vi "Lab3_FSK.vi"() -> ()   [LabVIEW 2019]
uses:
  <vilib>/addons/Modulation/Digital/General/MT Generate Bits (Galois, PN Order).vi
  <vilib>/addons/Modulation/Digital/Support/Common/Validators/mod_Generate Bits Validate.vi
  <vilib>/addons/Modulation/Analog/support/mod_Set Error Source.vi
  <vilib>/addons/Modulation/Digital/Support/Common/Validators/mod_AWGN Validate.vi
  <vilib>/addons/Modulation/Digital/Impairments/subVIs/mod_createSeeds.vi
  <vilib>/addons/Modulation/Digital/Support/Common/Validators/mod_Validate Samples Per Symbol.vi
  <vilib>/addons/Modulation/Analog/support/Validators/mod_Validate Complex Waveform.vi
  <vilib>/addons/Modulation/Analog/support/Validators/mod_WFErrorHandler.vi
  <vilib>/addons/Modulation/Digital/General/subVIs/mod_Generate Bits PN Sequence.vi
  <vilib>/addons/Modulation/Digital/General/MT Generate FSK System Parameters(M).vi
  <vilib>/Analysis/1siggen.llb/Gaussian White Noise (obs 90).vi
  <vilib>/addons/Modulation/Analog/MT Upconvert Baseband (Real).vi
  <vilib>/express/express analysis/Spectral/Block/exnSpectralBlock spectral measurements RMS poly.vi
  <vilib>/express/express analysis/Spectral/Block/exnSpectralBlock spectral measurements RMS DDT.vi
  <vilib>/express/express analysis/Spectral/XNode/ExpressSpectralMeasurementsBlockNode.xnode
  <vilib>/addons/Modulation/niDMT.lvlib
  <vilib>/addons/Modulation/niAMT.lvlib
panel:
  in  "stop 2":bool
  in  "Tab Control":enum32{"FFR(RMS)", "Module Signal"}(tab)
  out "FFR(RMS)":dynamicdata(graph)
  out "Module Signal":cluster{"t0":dbl, "dt":dbl, "Y":dbl[]}(graph)
  in  "FSK Derivation":dbl format="%#_2p"
  in  "Symbol (HZ)":dbl format="%#_2p"
  in  "Carrier Freq(HZ)":dbl format="%#_2p"
  in  "M-FSK":u16(ring) items=["2"=2, "4"=4, "8"=8, "16"=16]
  in  "Eb/No(dB)":dbl
  in  "stop":bool
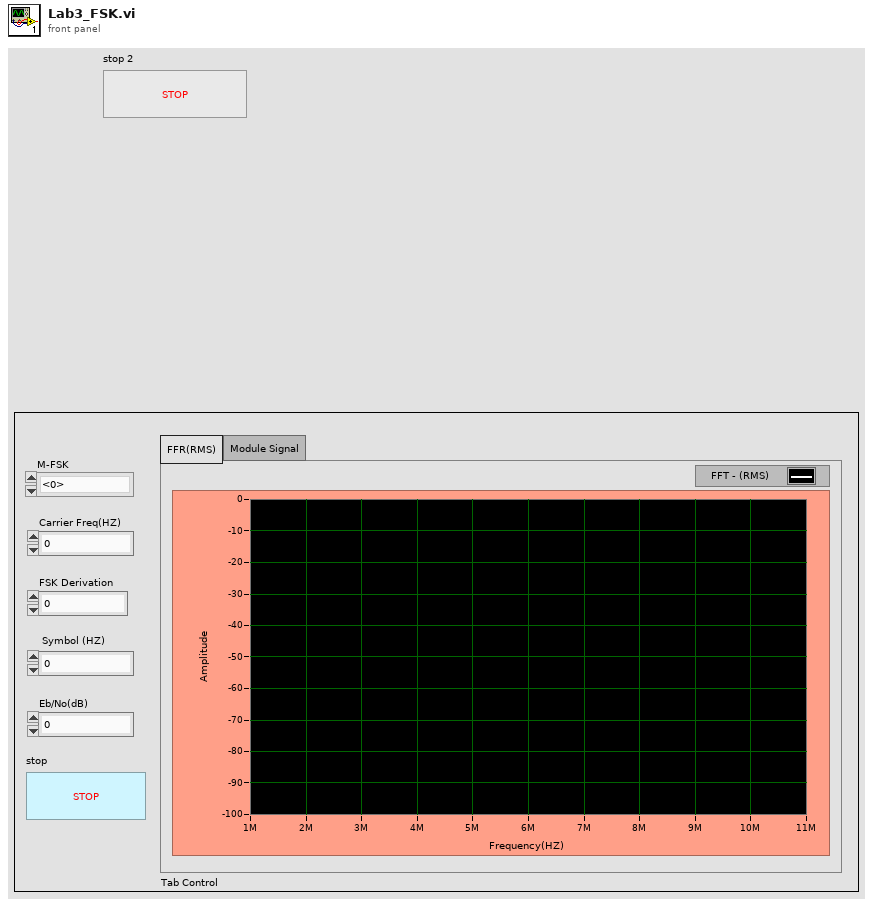
[diagram p1: front panel]
types:
  T1 = cluster{"averaging mode":u16, "weighting mode":u16, "number of averages":u32}
  T2 = cluster{"dB On (F)":bool, "unwrap phase (F)":bool, "convert to degree (F)":bool}
  T3 = cluster{"samples per symbol (16)":i32, "symbol map":dbl[], "symbol phase continuity":enum16{"continuous", "discontinuous"}}
  T4 = typedef "niAMT.lvlib/Complex Data Waveform.ctl" = cluster{"t0":dbl, "dt":dbl, "Y":cdb[]}
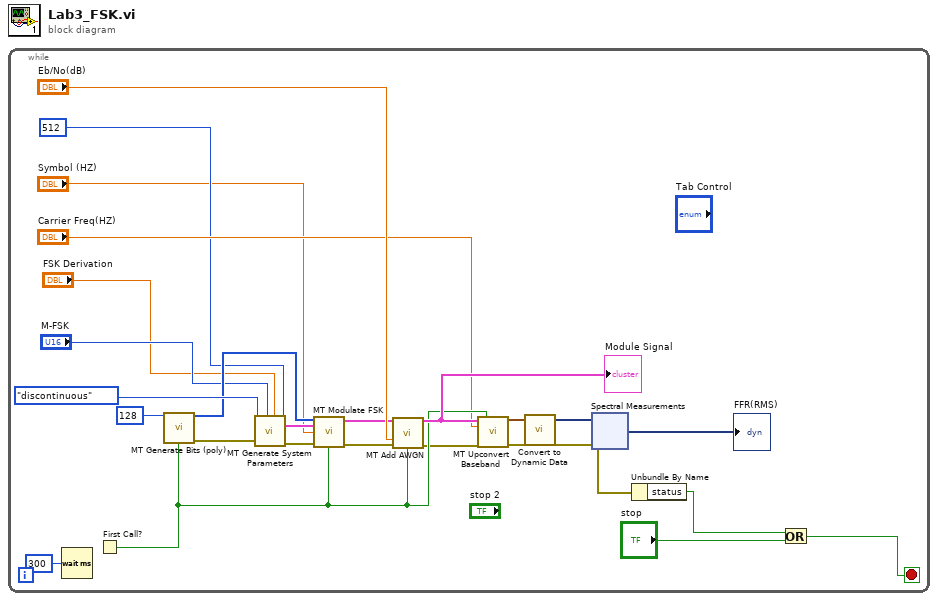
[diagram p0: block diagram]
diagram:
  n1 = while {
    stop <- w1 stop-if-true
    n2 = Wait (ms)(milliseconds to wait=u32 300) -> ()  [unwired: 1 out]
    n3 = First Call?() -> (First Call?: T/F=w19:bool)
    n4 = call-poly <vilib>:"MT Generate Bits (poly).vi"("total bits (128)"=128, "reset? (T)"=w19) -> ("output bit stream"=w11:i8[], "error out"=w18:errorcluster)  [unwired: 11 in, 1 out]
    n5 = call-poly <vilib>:"MT Generate System Parameters.vi"("samples per symbol (16)"=512, "M-FSK (2)"="M-FSK", "FSK deviation (Hz)"="FSK Derivation", "symbol phase continuity"=enum16{"continuous", "discontinuous"}."discontinuous", "error in (no error)"=w18) -> ("FSK system parameters"=w20:T3, "error out"=w17:errorcluster)  [unwired: 8 in, 1 out]
    n6 = call <vilib>:"MT Modulate FSK.vi"("input bit stream"=w11, "FSK system parameters"=w20, "symbol rate (Hz)"="Symbol (HZ)", "error in (no error)"=w17, "reset? (T)"=w19) -> ("output complex waveform"=w3:T4, "error out"=w16:errorcluster)  [unwired: 8 in, 1 out]
    n7 = call <vilib>:"MT Add AWGN.vi"("input complex waveform"=w3, "Eb/N0 (10 dB)"="Eb/No(dB)", "error in (no error)"=w16, "reset? (T)"=w19) -> ("output complex waveform"=w24:T4, "error out"=w15:errorcluster)  [unwired: 9 in, 1 out]
    "Module Signal" <- w24
    n8 = call-poly <vilib>:"MT Upconvert Baseband.vi"("baseband waveform (complex)"=w24, "reset? (F)"=w19, "carrier frequency (Hz)"="Carrier Freq(HZ)", "error in (no error)"=w15) -> ("passband waveform"=w12:waveform(dbl), "error out"=w14:errorcluster)  [unwired: 10 in]
    n9 = call "Convert to Dynamic Data"("Waveform"=w12) -> ("Dynamic Data Type"=w13:dynamicdata)  [unwired: 3 in]
    n10 = xnode "Spectral Measurements"("Signals"=w13, "error in (no error)"=w14) -> ("FFT - (RMS)"=→"FFR(RMS)":dynamicdata, "error out"=w21:errorcluster)  [unwired: 1 out]
    n11 = Unbundle By Name(w21) -> ("status"=w22:bool)
    n12 = Or(x=w22, y="stop") -> (x .or. y?=w1:bool)
  }
